vi "Tosca-Apply Rep Number Specific Scaling.vi"(0 "Waveform in":dbl[][](array[numeric]), 2 "State":i32, 5 "DO Array in":bool[][](array[boolean]), 11 "Max Nrep":i32, 12 "ramp off":bool[](array[boolean]), 13 "Rep #":i32) -> (4 "Waveform out":dbl[][](array[numeric]), 6 "DO Array out":bool[][](array[boolean]))   [LabVIEW 2020]
uses:
  Trace VIs/Tosca-Trace-Event.ctl
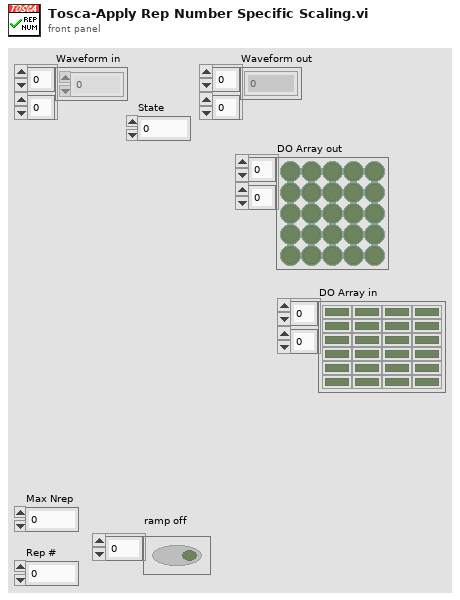
[diagram p1: front panel]
types:
  T1 = typedef "Tosca-Trace-Event.ctl" = enum16{"Unspecified", "Trial start", "Enqueue", "Result", "End parser", "Frame", "Queue available", "Timeout sent", "WritePos", "TTL"}
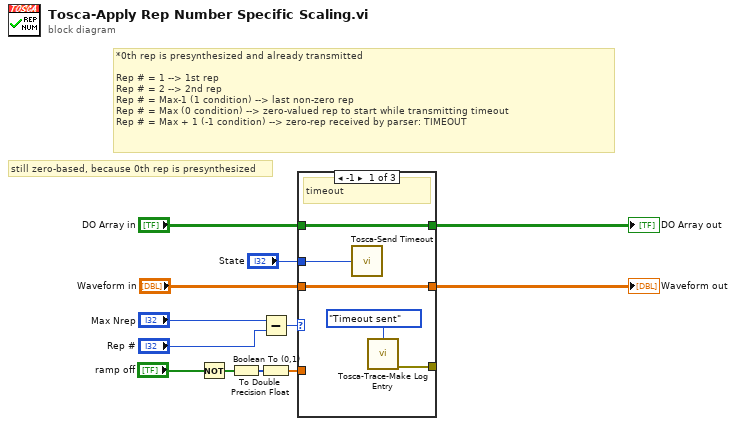
[diagram p0: block diagram]
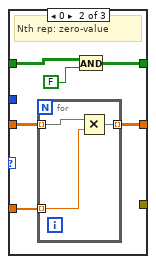
[diagram p2: hidden frame]
diagram:
  # "still zero-based, because 0th rep is presynthesized"
  # "*0th rep is presynthesized and already transmitted\n\nRep # = 1 --> 1st rep\nRep # = 2 --> 2nd rep \nRep # = Max-1 (1 condition) --> last non-zero rep\nRep # = Max (0 condition) --> zero-valued rep to start while transmitting timeout\nRep # = Max + 1 (-1 condition) --> zero-rep received by parser: TIMEOUT"
  n1 = Not(x="ramp off") -> (.not. x?=w5:bool[])
  n2 = Boolean To (0,1)(Boolean=w5) -> (0, 1=w4:i16[])
  n3 = Subtract(x="Max Nrep", y="Rep #") -> (x-y=w8:i32)
  n4 = To Double Precision Float(number=w4) -> (double precision float=w3:dbl[])
  n5 = case shown="-1" w8 {
    tunnel: "Waveform in" -> [w17 w23 w28]
    tunnel: [w17 w22 w28] -> w12
    tunnel: "DO Array in" -> [w16 w21 w27]
    tunnel: [w16 w20 w27] -> w11
    tunnel: w3 -> [_ w18 _]
    tunnel: "State" -> [w15 _ _]
    tunnel: [w13 _ _] -> _
    frame -1 {
      # "timeout"
      n6 = call "Tosca-Send Timeout.vi"("State"=w15) -> ()  [unwired: 15 in]
      n7 = call "Tosca-Trace-Make Log Entry.vi"("Event"=Tosca-Trace-Event."Timeout sent") -> ("error out"=w13:errorcluster)  [unwired: 14 in]
    }
    frame 0 {
      # "Nth rep: zero-value"
      n8 = for {
        tunnel: w23 -> [w26] mode=indexing
        tunnel: [w25] -> w22 mode=indexing
        tunnel: w18 -> [w24] mode=indexing
        n9 = Multiply(x=w26, y=w24) -> (x*y=w25:dbl[])
      }
      n10 = And(x=w21, y=FALSE) -> (x .and. y?=w20:bool[][])
    }
    frame 1, Default {
      # "Steady state"
    }
  }
  "Waveform out" <- w12
  "DO Array out" <- w11
